vi "GetTCSInfo.vi"() -> (0 "TCSInfo":T1)   [LabVIEW 2015]
uses:
  TCSLINK_global.vi
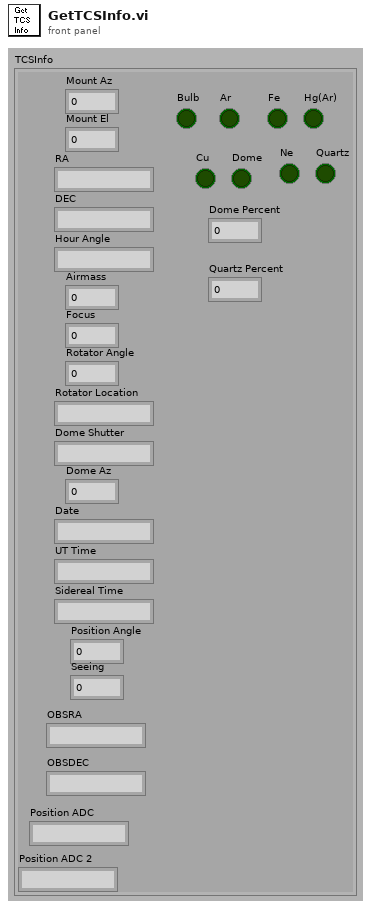
[diagram p1: front panel]
types:
  T1 = cluster{"Mount Az":dbl, "Mount El":dbl, "RA":string, "DEC":string, "Hour Angle":string, "Airmass":dbl, "Focus":dbl, "Rotator Angle":dbl, "Rotator Location":string, "Dome Shutter":string, "Dome Az":dbl, "Date":string, "UT Time":string, "Sidereal Time":string, "Position Angle":dbl, "Seeing":dbl, "OBSRA":string, "OBSDEC":string, "Position ADC":string, "Position ADC 2":string, "Bulb":bool, "Ar":bool, "Cu":bool, "Dome":bool, "Fe":bool, "Hg(Ar)":bool, "Ne":bool, "Quartz":bool, "Dome Percent":dbl, "Quartz Percent":dbl}
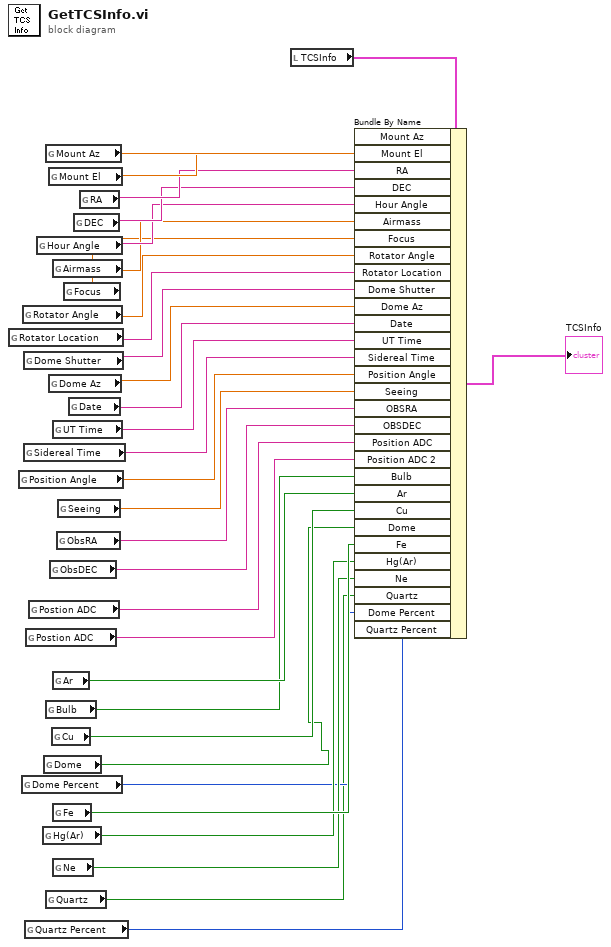
[diagram p0: block diagram]
diagram:
  n1 = global read "TCSLINK_global.vi" "Rotator Location"() -> (w24:string)
  n2 = global read "TCSLINK_global.vi" "Position Angle"() -> (w18:dbl)
  n3 = global read "TCSLINK_global.vi" "Dome Percent"() -> (w3:i8)
  n4 = global read "TCSLINK_global.vi" "Rotator Angle"() -> (w25:dbl)
  n5 = global read "TCSLINK_global.vi" "Dome Shutter"() -> (w23:string)
  n6 = global read "TCSLINK_global.vi" "Sidereal Time"() -> (w19:string)
  n7 = global read "TCSLINK_global.vi" "Quartz Percent"() -> (w4:i8)
  n8 = global read "TCSLINK_global.vi" "Postion ADC"() -> (w13:string)
  n9 = global read "TCSLINK_global.vi" "Postion ADC"() -> (w14:string)
  n10 = global read "TCSLINK_global.vi" "Hour Angle"() -> (w28:string)
  n11 = global read "TCSLINK_global.vi" "Hg(Ar)"() -> (w6:bool)
  n12 = global read "TCSLINK_global.vi" "Dome"() -> (w11:bool)
  n13 = global read "TCSLINK_global.vi" "Mount Az"() -> (w32:dbl)
  n14 = global read "TCSLINK_global.vi" "Bulb"() -> (w8:bool)
  n15 = global read "TCSLINK_global.vi" "Quartz"() -> (w1:bool)
  n16 = global read "TCSLINK_global.vi" "Mount El"() -> (w31:dbl)
  n17 = global read "TCSLINK_global.vi" "Dome Az"() -> (w22:dbl)
  n18 = global read "TCSLINK_global.vi" "ObsDEC"() -> (w15:string)
  n19 = global read "TCSLINK_global.vi" "Cu"() -> (w12:bool)
  n20 = global read "TCSLINK_global.vi" "Airmass"() -> (w27:dbl)
  n21 = global read "TCSLINK_global.vi" "UT Time"() -> (w20:string)
  n22 = global read "TCSLINK_global.vi" "Ar"() -> (w9:bool)
  n23 = global read "TCSLINK_global.vi" "Fe"() -> (w7:bool)
  n24 = global read "TCSLINK_global.vi" "Ne"() -> (w5:bool)
  n25 = global read "TCSLINK_global.vi" "ObsRA"() -> (w16:string)
  n26 = global read "TCSLINK_global.vi" "Seeing"() -> (w17:dbl)
  n27 = global read "TCSLINK_global.vi" "Focus"() -> (w26:dbl)
  n28 = global read "TCSLINK_global.vi" "Date"() -> (w21:string)
  n29 = global read "TCSLINK_global.vi" "DEC"() -> (w29:string)
  n30 = global read "TCSLINK_global.vi" "RA"() -> (w30:string)
  n31 = local read "TCSInfo"() -> (w10:T1)
  n32 = Bundle By Name(cluster=w10, "Mount Az"=w32, "Mount El"=w31, "RA"=w30, "DEC"=w29, "Hour Angle"=w28, "Airmass"=w27, "Focus"=w26, "Rotator Angle"=w25, "Rotator Location"=w24, "Dome Shutter"=w23, "Dome Az"=w22, "Date"=w21, "UT Time"=w20, "Sidereal Time"=w19, "Position Angle"=w18, "Seeing"=w17, "OBSRA"=w16, "OBSDEC"=w15, "Position ADC"=w14, "Position ADC 2"=w13, "Bulb"=w8, "Ar"=w9, "Cu"=w12, "Dome"=w11, "Fe"=w7, "Hg(Ar)"=w6, "Ne"=w5, "Quartz"=w1, "Dome Percent"=w3, "Quartz Percent"=w4) -> (→"TCSInfo":T1)
